vi "Validate Variable Header.vi"(8 "error in (no error)":errorcluster, 11 "CONNECT in":refnum<class "CONNECT.lvclass">) -> (0 "error out":errorcluster, 1 "valid?":bool, 3 "CONNECT out":refnum<class "CONNECT.lvclass">)   [LabVIEW 2013, in "CONNECT.lvclass"]
uses:
  CONNECT.lvclass
  ControlPacket/ControlPacket.lvclass/ControlPacket.ctl
  ControlPacket/ControlPacket.lvclass
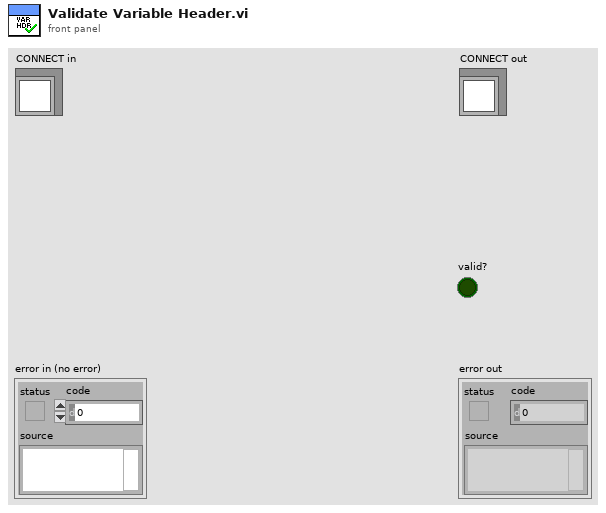
[diagram p1: front panel]
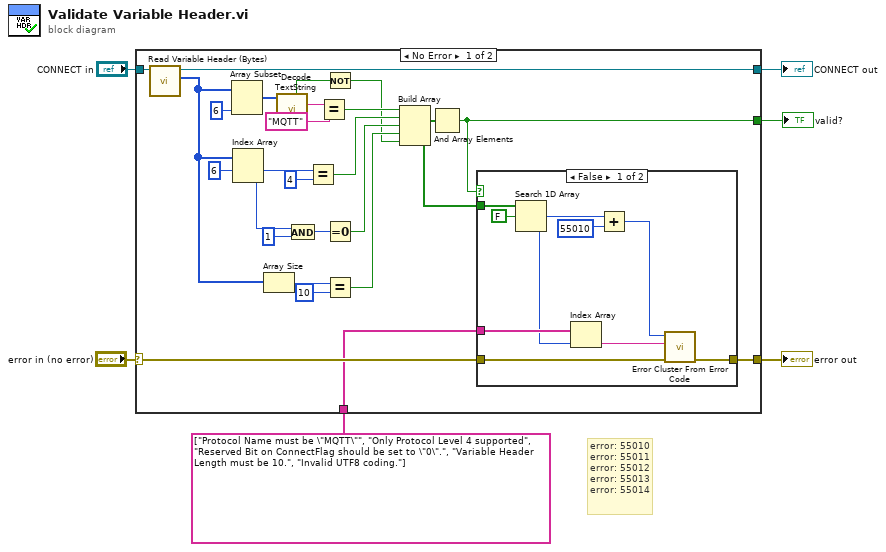
[diagram p0: block diagram]
diagram:
  # "error: 55010\nerror: 55011\nerror: 55012\nerror: 55013\nerror: 55014"
  n1 = case shown="No Error" "error in (no error)" {
    selector: "error in (no error)" -> [w16 w43]
    tunnel: "CONNECT in" -> [w32 w44]
    tunnel: [w31 w44] -> w5
    tunnel: [w11 _] -> w4
    tunnel: [w17 w43] -> w3
    tunnel: string[] ["Protocol Name must be \"MQTT\"", "Only Protocol Level 4 supported", "Reserved Bit on ConnectFlag should be set to \"0\".", "Variable Header Length must be 10.", "Invalid UTF8 coding."] -> [w9 _]
    frame No Error {
      n2 = call "Read Variable Header (Bytes).vi"("ControlPacket in"=w32) -> ("Variable Header (Bytes)"=w20:u8[], "ControlPacket out"=w31:refnum<class "CONNECT.lvclass">)  [unwired: 9 in]
      n3 = Array Subset(array=w20, length=6) -> (w29:u8[])  [unwired: 1 in]
      n4 = Index Array(array=w20, index #1=6 ("index")) -> (element #1=w25:u8, element #2=w23:u8)  [unwired: 1 in]
      n5 = Array Size(array=w20) -> (size(s)=w19:i32)
      n6 = call "Decode TextString.vi"("Length-Prefixed Field"=w29) -> ("Text String"=w28:string, "restricted code"=w8:bool)  [unwired: 8 in, 1 out]
      n7 = And(x=w23, y=u8 1) -> (x .and. y?=w21:u8)
      n8 = Equal?(x=w25, y=u8 4) -> (x = y?=w14:bool)
      n9 = Equal?(x=w28, y="MQTT") -> (x = y?=w15:bool)
      n10 = Not(x=w8) -> (.not. x?=w7:bool)
      n11 = Equal To 0?(x=w21) -> (x = 0?=w13:bool)
      n12 = Equal?(x=w19, y=10) -> (x = y?=w12:bool)
      n13 = Build Array(w15, w14, w13, w12, w7) -> (w10:bool[])
      n14 = And Array Elements(Boolean array=w10) -> (logical AND=w11:bool)
      n15 = case shown="False" w11 {
        tunnel: w16 -> [w40 w42]
        tunnel: [w41 w42] -> w17
        tunnel: w10 -> [w39 _]
        tunnel: w9 -> [w37 _]
        frame False {
          n16 = Search 1D Array(1D array=w39, element=FALSE) -> (index of element=w35:i32)  [unwired: 1 in]
          n17 = Index Array(array=w37, index=w35) -> (element=w36:string)
          n18 = Add(x=w35, y=55010 ("error code (0)")) -> (x+y=w33:i32)
          n19 = call <vilib>:"Error Cluster From Error Code.vi"("error in (no error)"=w40, "error message (\"\")"=w36, "error code (0)"=w33) -> ("error out"=w41:errorcluster)  [unwired: 6 in]
        }
        frame True {
        }
      }
    }
    frame Error {
    }
  }
  "error out" <- w3
  "CONNECT out" <- w5
  "valid?" <- w4
